vi "Get Engine.vi"(0 "Application Manager In":refnum<k7>, 1 "error in (no error)":errorcluster) -> (2 "Application Manager Out":refnum<k7>, 3 "TestStand Engine":refnum<k7>, 4 "error out":errorcluster)   [LabVIEW 2010, in "TS Simple LabVIEW OI Dependencies.lvlib"]
uses:
  TS Simple LabVIEW OI Dependencies.lvlib
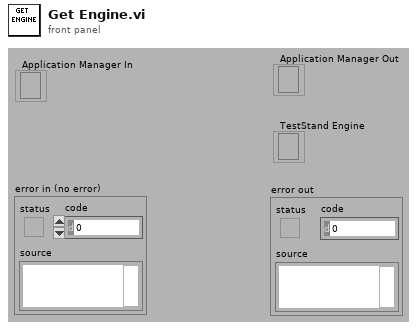
[diagram p1: front panel]
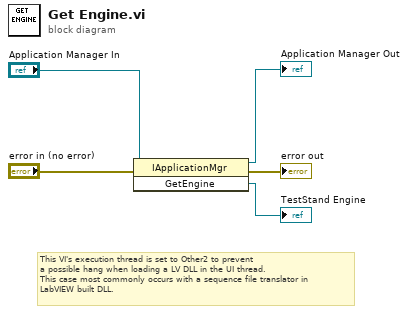
[diagram p0: block diagram]
diagram:
  # "This VI's execution thread is set to Other2 to prevent\na possible hang when loading a LV DLL in the UI thread.\nThis case most commonly occurs with a sequence file translator in\nLabVIEW built DLL."
  n1 = invoke class="IApplicationMgr" method="GetEngine"(reference="Application Manager In", error in="error in (no error)") -> (reference out=→"Application Manager Out":refnum<k7>, error out=→"error out":errorcluster, "GetEngine"=→"TestStand Engine":refnum<k7>)  [unwired: 1 in]
